vi "AOTF_Create_analog_Ports.vi"() -> (1 "task out":refnum<k21>, 2 "error out":errorcluster)   [LabVIEW 2011]
uses:
  <vilib>/DAQmx/create/channels.llb/DAQmx Create Channel (AO-Voltage-Basic).vi
panel:
  in  "physical channels 7":tag
  in  "physical channels 6":tag
  in  "physical channels 5":tag
  in  "physical channels 4":tag
  in  "physical channels 3":tag
  in  "physical channels 2":tag
  in  "physical channels 1":tag
  in  "physical channels":tag
  in  "error in":errorcluster
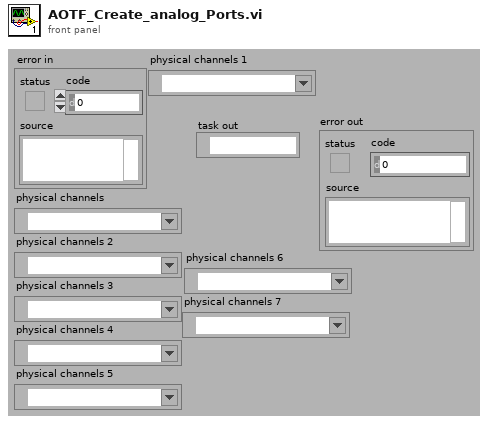
[diagram p1: front panel]
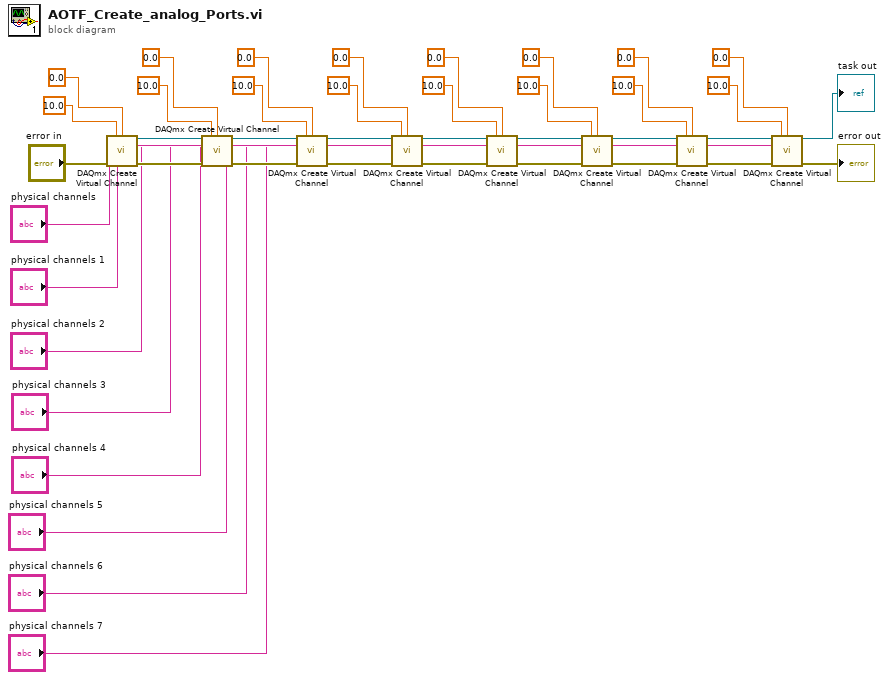
[diagram p0: block diagram]
diagram:
  n1 = call-poly <vilib>:"DAQmx Create Virtual Channel.vi"("maximum value"=10.0, "minimum value"=0.0, "physical channels"="physical channels", "error in"="error in") -> ("task out"=w39:refnum<k21>, "error out"=w38:errorcluster)  [unwired: 5 in, 5 out]
  n2 = call-poly <vilib>:"DAQmx Create Virtual Channel.vi"("task in"=w39, "maximum value"=10.0, "minimum value"=0.0, "physical channels"="physical channels 1", "error in"=w38) -> ("task out"=w36:refnum<k21>, "error out"=w37:errorcluster)  [unwired: 4 in, 5 out]
  n3 = call-poly <vilib>:"DAQmx Create Virtual Channel.vi"("task in"=w36, "maximum value"=10.0, "minimum value"=0.0, "physical channels"="physical channels 2", "error in"=w37) -> ("task out"=w34:refnum<k21>, "error out"=w35:errorcluster)  [unwired: 4 in, 5 out]
  n4 = call-poly <vilib>:"DAQmx Create Virtual Channel.vi"("task in"=w34, "maximum value"=10.0, "minimum value"=0.0, "physical channels"="physical channels 3", "error in"=w35) -> ("task out"=w33:refnum<k21>, "error out"=w32:errorcluster)  [unwired: 4 in, 5 out]
  n5 = call-poly <vilib>:"DAQmx Create Virtual Channel.vi"("task in"=w33, "maximum value"=10.0, "minimum value"=0.0, "physical channels"="physical channels 4", "error in"=w32) -> ("task out"=w26:refnum<k21>, "error out"=w27:errorcluster)  [unwired: 4 in, 5 out]
  n6 = call-poly <vilib>:"DAQmx Create Virtual Channel.vi"("task in"=w26, "maximum value"=10.0, "minimum value"=0.0, "physical channels"="physical channels 5", "error in"=w27) -> ("task out"=w28:refnum<k21>, "error out"=w29:errorcluster)  [unwired: 4 in, 5 out]
  n7 = call-poly <vilib>:"DAQmx Create Virtual Channel.vi"("task in"=w28, "maximum value"=10.0, "minimum value"=0.0, "physical channels"="physical channels 6", "error in"=w29) -> ("task out"=w30:refnum<k21>, "error out"=w31:errorcluster)  [unwired: 4 in, 5 out]
  n8 = call-poly <vilib>:"DAQmx Create Virtual Channel.vi"("task in"=w30, "maximum value"=10.0, "minimum value"=0.0, "physical channels"="physical channels 7", "error in"=w31) -> ("task out"=→"task out":refnum<k21>, "error out"=→"error out":errorcluster)  [unwired: 4 in, 5 out]
